vi "KE2425_Acquire.vi"(6 "KeepOn?":bool=TRUE, 7 "Type":u16(ring) items=["First", "Second", "Init"], 8 "error in (no error)":errorcluster, 11 "Instruments in":refnum<class "Instruments.lvclass">) -> (0 "error out":errorcluster, 3 "Instruments out":refnum<class "Instruments.lvclass">, 4 "Keithley":bool, 5 "Voltage":dbl)   [LabVIEW 2012, in "Instruments.lvclass"]
uses:
  Instruments.lvclass
  Instruments.lvclass/Instruments.ctl
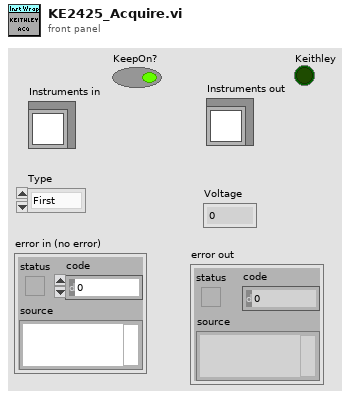
[diagram p1: front panel]
types:
  T1 = typedef "SMUParam.ctl" = cluster{"Start Current,mA":dbl, "Stop Current,mA":dbl, "Voltage Compliance,V":dbl, "GPIB":string, "VISA resource name":refnum<visa-resource-name>}
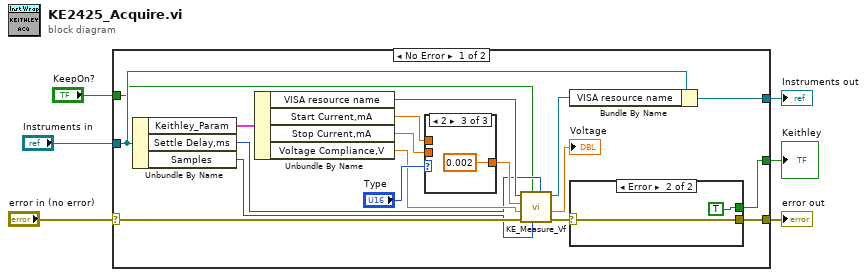
[diagram p0: block diagram]
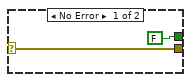
[diagram p2: hidden frame]
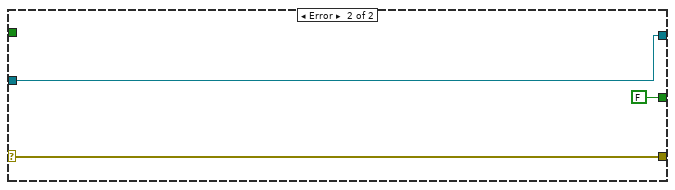
[diagram p5: hidden frame]
diagram:
  n1 = case shown="No Error" "error in (no error)" {
    selector: "error in (no error)" -> [w17 w34]
    tunnel: [w9 w34] -> w5
    tunnel: [w11 w33] -> w3
    tunnel: "Instruments in" -> [w14 w33]
    tunnel: "KeepOn?" -> [w7 _]
    tunnel: [w8 FALSE] -> w1
    frame No Error {
      n2 = Unbundle By Name(w14) -> ("Keithley_Param"=w21:T1, "Settle Delay,ms"=w16:u32, "Samples"=w15:i32)
      n3 = Unbundle By Name(w21) -> ("VISA resource name"=w18:refnum<visa-resource-name>, "Start Current,mA"=w23:dbl, "Stop Current,mA"=w22:dbl, "Voltage Compliance,V"=w19:dbl)
      n4 = case shown="2" "Type" {
        tunnel: w23 -> [w29 _ _]
        tunnel: w22 -> [_ w30 _]
        tunnel: [w29 w30 0.002 ("Stop Current,mA")] -> w20
        frame 0, Default {
        }
        frame 1 {
        }
        frame 2 {
        }
      }
      n5 = call "KE_Measure_Vf.vi"("Settle Delay"=w16, "Samples"=w15, "Keep On"=w7, "error in (no error)"=w17, "Compliance"=w19, "Current(A)"=w20, "KE_In"=w18) -> ("error out"=w10:errorcluster, "Vf"=→"Voltage":dbl, "KE_Out"=w13:refnum<visa-resource-name>)  [unwired: 2 in]
      n6 = Bundle By Name(cluster=w14, "VISA resource name"=w13) -> (w11:refnum<class "Instruments.lvclass">)
      n7 = case shown="Error" w10 {
        selector: w10 -> [w25 w27]
        tunnel: [FALSE TRUE] -> w8
        tunnel: [w25 w27] -> w9
        frame No Error {
        }
        frame Error {
        }
      }
    }
    frame Error {
    }
  }
  "error out" <- w5
  "Instruments out" <- w3
  "Keithley" <- w1
